vi "aFGV - License Read Write RT.vi"(6 "State":enum16{"Read", "Write"}(ring), 8 "Error In":errorcluster, 10 "Path":path, 11 "Data In":T1={"Expired Time"="", "Serial Number"="", "Product Name"="", "Period"=0, "Activated Time"="", "License Level"=enum."Level 1", "License Type"=enum."Trial", "Log Time"=""}) -> (0 "Error Out":errorcluster, 3 "Data Out":T1={"Expired Time"="", "Serial Number"="", "Product Name"="", "Period"=0, "Activated Time"="", "License Level"=enum."Level 1", "License Type"=enum."Trial", "Log Time"=""})   [LabVIEW 2020]
uses:
  Control/License File Parameter RT.ctl
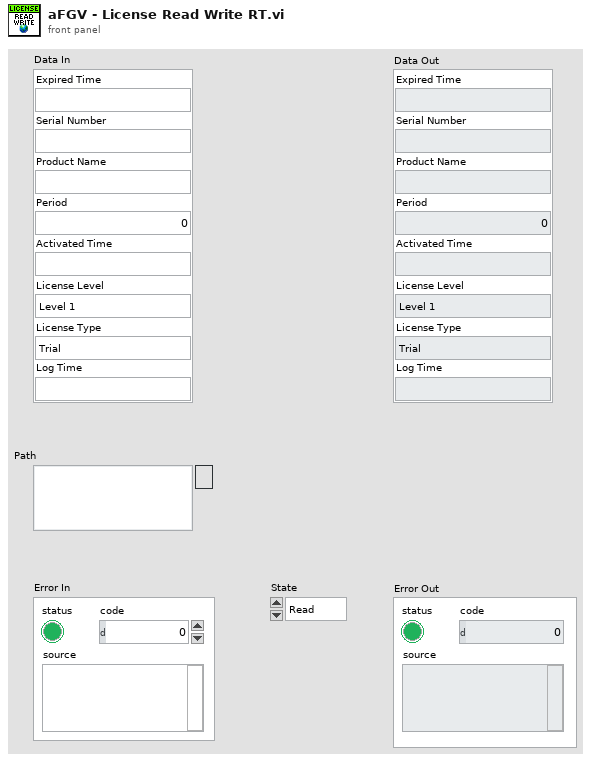
[diagram p1: front panel]
types:
  T1 = typedef "License File Parameter RT.ctl" = cluster{"Expired Time":string, "Serial Number":string, "Product Name":string, "Period":i16, "Activated Time":string, "License Level":enum16{"Level 1", "Level 2", "Level 3", "Level 4", "Level 5"}, "License Type":enum16{"Free", "Trial", "Subscription", "Perpetual"}, "Log Time":string}
  T2 = enum16{"open", "replace", "create", "open or create", "replace or create", "replace or create with confirmation"}
  T3 = enum16{"big-endian, network order", "native, host order", "little-endian"}
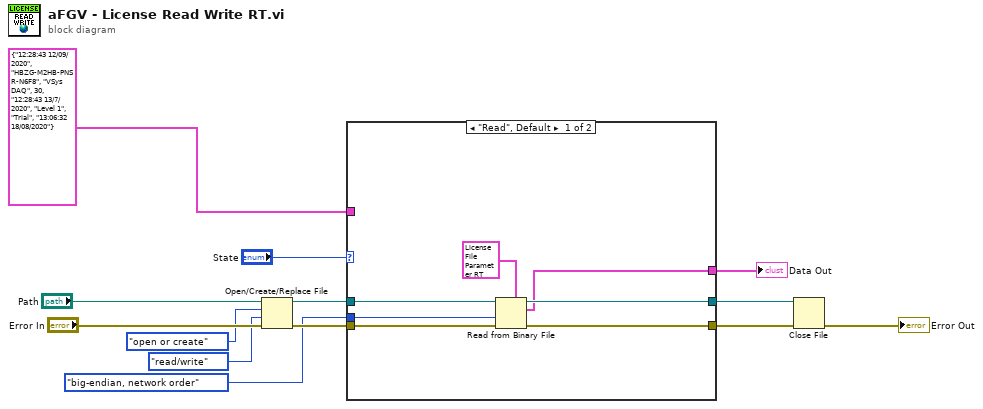
[diagram p0: block diagram]
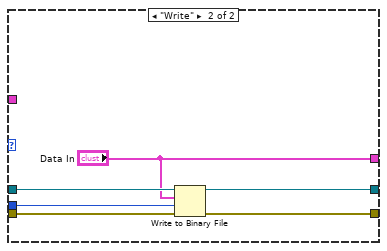
[diagram p2: hidden frame]
diagram:
  n1 = Open/Create/Replace File(file path (use dialog)="Path", error in="Error In", operation (0:open)=T2."open or create", access (0:read/write)=enum16{"read/write", "read-only", "write-only"}."read/write") -> (refnum out=w5:refnum<file>, error out=w10:errorcluster)  [unwired: 2 in, 1 out]
  n2 = case shown="\"Read\", Default" "State" {
    tunnel: [w20 w25] -> w11
    tunnel: w10 -> [w19 w26]
    tunnel: [w18 w23] -> w9
    tunnel: T3."big-endian, network order" ("byte order") -> [w17 w24]
    tunnel: w5 -> [w16 w22]
    tunnel: [w14 "Data In"] -> w2
    tunnel: T1 {"Expired Time"="12:28:43 12/09/2020", "Serial Number"="HBZG-M2HB-PNSR-N6F8", "Product Name"="VSys DAQ", "Period"=30, "Activated Time"="12:28:43 13/7/2020", "License Level"=enum."Level 1", "License Type"=enum."Trial", "Log Time"="13:06:32 18/08/2020"} ("Data In 2") -> [_ _]
    frame "Read", Default {
      n3 = Read from Binary File(5:T1 {"Expired Time"="", "Serial Number"="", "Product Name"="", "Period"=0, "Activated Time"="", "License Level"=enum."Level 1", "License Type"=enum."Trial", "Log Time"=""} ("License File Param"), 8:w19, 9:w17, 11:w16) -> (0:w20:errorcluster, 2:w14:T1, 3:w18:refnum<file>)  [unwired: 2 in, 1 out]
    }
    frame "Write" {
      n4 = Write to Binary File(file (use dialog)=w22, data="Data In", error in=w26, 9:w24) -> (refnum out=w23:refnum<file>, error out=w25:errorcluster)  [unwired: 2 in, 1 out]
    }
  }
  "Data Out" <- w2
  n5 = Close File(refnum=w9, error in=w11) -> (error out=→"Error Out":errorcluster)  [unwired: 1 out]
